vi "demo.vi"() -> ()   [LabVIEW 2014]
panel:
  out "return type":dbl
  in  "x":dbl=2.0
  in  "y":dbl=1.0
  in  "Combo Box":string(combo)
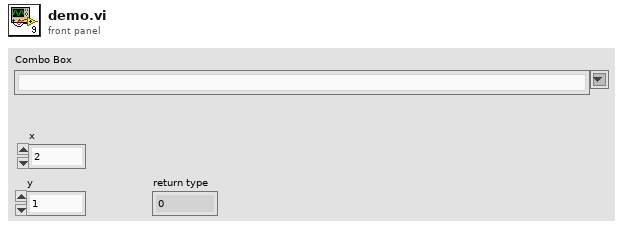
[diagram p1: front panel]
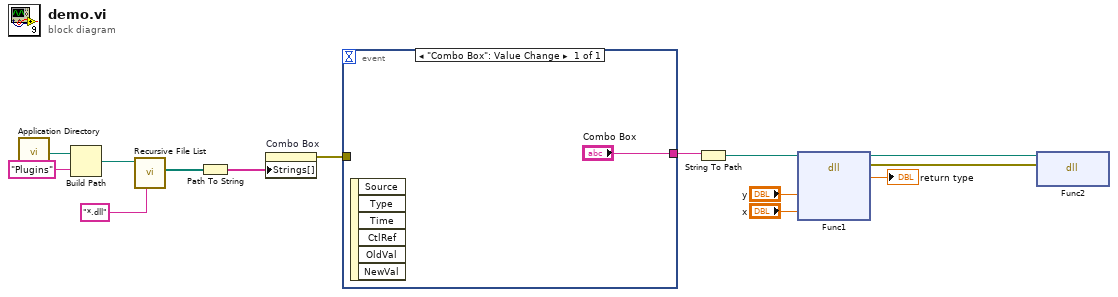
[diagram p0: block diagram]
diagram:
  n1 = call <vilib>:"Application Directory.vi"() -> ("Application Directory"=w14:path)
  n2 = Build Path(base path=w14, name or relative path="Plugins") -> (appended path=w12:path)
  n3 = call <vilib>:"Recursive File List.vi"("pattern"="*.dll", "Folder Path"=w12) -> ("All Files in Dir"=w10:path[])  [unwired: 5 in, 4 out]
  n4 = Path To String(path=w10) -> (string=w9:string[])
  n5 = property on="Combo Box" class="CmbBox"("Strings[]"=w9) -> (error out=w8:errorcluster)  [unwired: 2 in, 1 out]
  n6 = event shown="[0] \"Combo Box\": Value Change" {
    selector: _ -> [_]
    dyn-events: _ -> [_]
    timeout: _ -> [_]
    tunnel: w8 -> [_]
    tunnel: ["Combo Box"] -> w7
    event "Combo Box": Value Change {
      n7 = event-data() -> ()  [unwired: 1 in, 6 out]
    }
  }
  n8 = String To Path(string=w7) -> (path=w4:path)
  n9 = dll-call lib="D:/Projects/LabVIEW-Design-Pattern/Plugin Template/dll/Plugin Template.dll" fn="Func1"(path in=w4, "y"="y", "x"="x") -> (path out=w5:path, error out=w6:errorcluster, "return type"=→"return type":dbl)  [unwired: 4 in]
  n10 = dll-call lib="D:/Projects/LabVIEW-Design-Pattern/Plugin Template/dll/Plugin Template.dll" fn="Func2"(path in=w5, error in=w6) -> ()  [unwired: 2 in, 2 out]
